vi "ProportionalSpeedControl.vi"(8 "Maximum Rate":dbl, 9 "Proportional Constant":dbl, 10 "Encoder Rate":dbl, 11 "Target":dbl) -> (3 "Output":dbl)   [LabVIEW 2014]
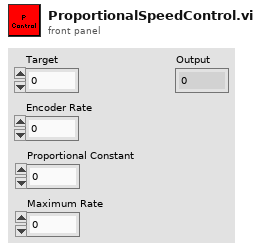
[diagram p1: front panel]
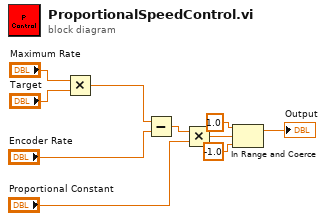
[diagram p0: block diagram]
diagram:
  n1 = Multiply(x="Maximum Rate", y="Target") -> (x*y=w1:dbl)
  n2 = Subtract(x=w1, y="Encoder Rate") -> (x-y=w5:dbl)
  n3 = Multiply(x=w5, y="Proportional Constant") -> (x*y=w9:dbl)
  n4 = In Range and Coerce(upper limit=1.0, x=w9, lower limit=-1.0) -> (coerced(x)=→"Output":dbl)  [unwired: 1 out]
